vi "Clean.vi"(0 "SourceDist_LV in":refnum<class "SourceDist_LV.lvclass">) -> (4 "SourceDist_LV out":refnum<class "SourceDist_LV.lvclass">)   [LabVIEW 2017, in "CL_G3_VIComponentBuilder.lvlib" / "SourceDist_LV.lvclass"]
doc: "Removes this export from the build machine."
uses:
  SourceDist_LV.lvclass
  C:/Tool Chain Support/Software Module Builder/Source/Exports/Exports/Export.lvclass
  C:/Tool Chain Support/Software Module Builder/Source/Exports/NI Build Specification_LV/NI Build Specification_LV.lvclass
  Exports/Export.lvclass/Export.ctl
  NI Build Specification_LV/NI Build Specification_LV.lvclass/NI Build Specification_LV.ctl
  Exports/Accessors/Read Export Operation Errors.vi
  Exports/Accessors/Read Component Export Dir.vi
  NI Build Specification_LV/Accessors/Read Export's Build Spec Name.vi
  NI Build Specification_LV/NI Build Specification_LV.lvclass
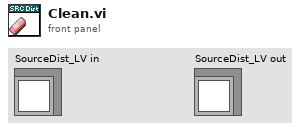
[diagram p1: front panel]
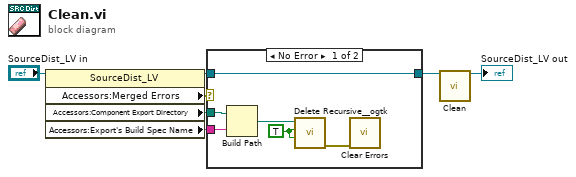
[diagram p0: block diagram]
diagram:
  n1 = property class="SourceDist_LV"(reference="SourceDist_LV in") -> (reference out=w4:refnum<class "SourceDist_LV.lvclass">, "Accessors:Merged Errors"=w5:errorcluster, "Accessors:Component Export Directory"=w2:path, "Accessors:Export's Build Spec Name"=w1:string)  [unwired: 1 in, 1 out]
  n2 = case shown="No Error" w5 {
    tunnel: w2 -> [w10 _]
    tunnel: [w12 w14] -> w3
    tunnel: w4 -> [w12 w14]
    tunnel: w1 -> [w11 _]
    frame No Error {
      w13 = TRUE ("Recursive? (FALSE)")
      n3 = Build Path(base path=w10, name or relative path=w11) -> (appended path=w9:path)
      n4 = call <userlib>:"Delete Recursive__ogtk.vi"("Ignore Read-Only? (FALSE)"=w13, "Recursive? (FALSE)"=w13, "Path"=w9) -> ("error out"=w8:errorcluster)  [unwired: 7 in, 1 out]
      n5 = call <vilib>:"Clear Errors.vi"("error in (no error)"=w8) -> ()  [unwired: 5 in, 2 out]
    }
    frame Error {
    }
  }
  n6 = call-parent "Clean.vi"("NI Build Specification_LV in"=w3) -> ("NI Build Specification_LV out"=→"SourceDist_LV out":refnum<class "SourceDist_LV.lvclass">)  [unwired: 14 in]
